vi "N-Create.vi"(8 "error in":errorcluster, 11 "Q Name":string) -> (0 "error out":errorcluster)   [LabVIEW 2016]
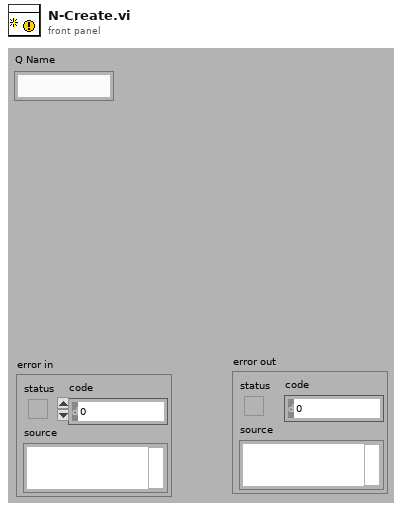
[diagram p1: front panel]
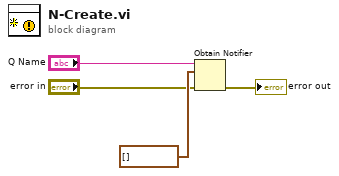
[diagram p0: block diagram]
diagram:
  n1 = Obtain Notifier(name (unnamed)="Q Name", notification data type=waveform(dbl)[] [] ("Waveform"), error in (no error)="error in") -> (error out=→"error out":errorcluster)  [unwired: 1 in, 2 out]
